vi "1B.5-Spoof Graph.vi"(1 "XY Graph":T1(array[cluster]), 2 "New Position":cluster{"X Position":dbl, "Y Position":dbl}) -> (0 "Array":cluster{"X Position":dbl, "Y Position":dbl}[](array[cluster]))   [LabVIEW 2011]
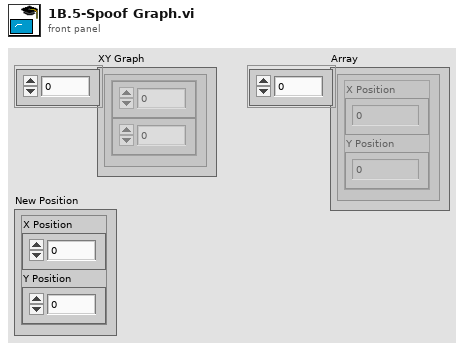
[diagram p1: front panel]
types:
  T1 = cluster{"Numeric Control":dbl, "Numeric Control":dbl}[]
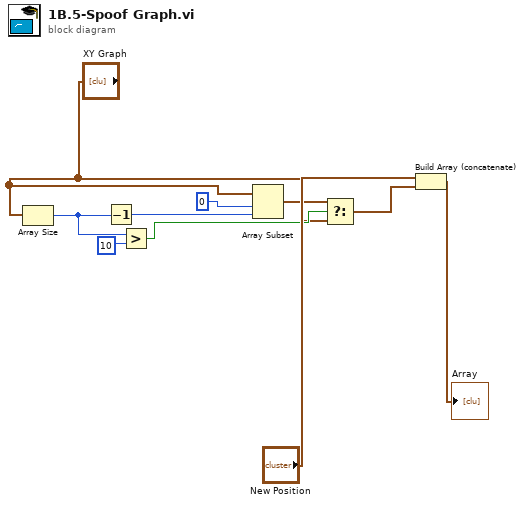
[diagram p0: block diagram]
diagram:
  n1 = Array Size(array="XY Graph") -> (size(s)=w7:i32)
  n2 = Decrement(x=w7) -> (x-1=w4:i32)
  n3 = Greater?(x=w7, y=10) -> (0:w9:bool)
  n4 = Array Subset(array="XY Graph", index=0, length=w4) -> (w6:T1)
  n5 = Select(t=w6, s=w9, f="XY Graph") -> (s? t:f=w1:T1)
  n6 = Build Array (concatenate)("New Position", w1) -> (→"Array":T1)
